vi "ADAM 5000 Get Voltages.vi"(8 "error in (no error)":errorcluster, 10 "AI Sensor Data":T1={"Sensor Array"=[{"Description"="P2 - LOX Tank Pressure", "Last Reading"="-124.89", "Coefs"=[-124.82, 244.17], "Eng Units"="psig"}, {"Description"="P3 - Fuel Tank Pressure", "Last Reading"="-124.89", "Coefs"=[-124.82, 244.17], "Eng Units"="psig"}, {"Description"="P1 - Chamber Pressure", "Last Reading"="-63.46", "Coefs"=[-63.442, 124.53], "Eng Units"="psig"}, {"Description"="Not Used", "Last Reading"="0.00", "Coefs"=[0.0, 0.0], "Eng Units"="psig"}, {"Description"="P5- DOME Reg.", "Last Reading"="-65.11", "Coefs"=[-65.132, -121.72], "Eng Units"="psig"}, {"Description"="Not Use", "Last Reading"="0.00", "Coefs"=[0.0, 0.0], "Eng Units"="psig"}, {"Description"="Load Cell", "Last Reading"="-6.72", "Coefs"=[-8.51, -8297.0], "Eng Units"="lb"}, {"Description"="P7 - Gnd High Pressure", "Last Reading"="-2.33", "Coefs"=[0.0, 10000.0], "Eng Units"="psig"}, {"Description"="High Press PT", "Last Reading"="-475.05", "Coefs"=[-483.6, 1244.5], "Eng Units"="psig"}, {"Description"="Dome Reg PT", "Last Reading"="-125.68", "Coefs"=[-126.9, 250.13], "Eng Units"="psig"}, {"Description"="FUEL PT", "Last Reading"="-125.44", "Coefs"=[-126.89, 250.01], "Eng Units"=""}, {"Description"="LOX PT", "Last Reading"="-128.32", "Coefs"=[-129.55, 251.63], "Eng Units"=""}, {"Description"="Chamber PT", "Last Reading"="-62.72", "Coefs"=[-63.442, 124.53], "Eng Units"=""}, {"Description"="LOX MV PT", "Last Reading"="-63.10", "Coefs"=[-63.711, 124.59], "Eng Units"=""}, {"Description"="FUEL MV PT", "Last Reading"="-61.90", "Coefs"=[-62.615, 123.79], "Eng Units"=""}, {"Description"="", "Last Reading"="0.00", "Coefs"=[0.0, 0.0], "Eng Units"=""}, {"Description"="Load Cell 0", "Last Reading"="-17.61", "Coefs"=[0.0, 16730.0], "Eng Units"=""}, {"Description"="Load Cell 1", "Last Reading"="13.17", "Coefs"=[0.0, 16730.0], "Eng Units"=""}, {"Description"="Load Cell 3", "Last Reading"="7.43", "Coefs"=[0.0, 16730.0], "Eng Units"=""}, {"Description"="Main Valve Closed Indicator", "Last Reading"="-0.00", "Coefs"=[0.0, 1.0], "Eng Units"="On/Off"}, {"Description"="Load Cell 1 - Veh Gross Weight", "Last Reading"="-125.78", "Coefs"=[-122.0, 8333.3], "Eng Units"="lbf"}, {"Description"="Load Cell 2 - - Veh Gross Weight", "Last Reading"="-3.62", "Coefs"=[0.0, 8333.33], "Eng Units"="lbf"}, {"Description"="Extra PT", "Last Reading"="-72.30", "Coefs"=[-72.241, 126.92], "Eng Units"=""}, {"Description"="Not Used", "Last Reading"="0.00", "Coefs"=[0.0, 0.0], "Eng Units"=""}, {"Description"="P6 - GHE Fill Pressure", "Last Reading"="-1035.38", "Coefs"=[-1035.0, 1261.6], "Eng Units"="psi"}, {"Description"="", "Last Reading"="0.00", "Coefs"=[], "Eng Units"=""}, {"Description"="", "Last Reading"="0.00", "Coefs"=[], "Eng Units"=""}, {"Description"="", "Last Reading"="0.00", "Coefs"=[], "Eng Units"=""}, {"Description"="", "Last Reading"="0.00", "Coefs"=[], "Eng Units"=""}, {"Description"="", "Last Reading"="0.00", "Coefs"=[], "Eng Units"=""}, {"Description"="", "Last Reading"="0.00", "Coefs"=[], "Eng Units"=""}, {"Description"="", "Last Reading"="0.00", "Coefs"=[], "Eng Units"=""}]}, 11 "Remote IP Address 2":string="192.168.10.200") -> (0 "error out":errorcluster, 1 "Slave Input Registers 2":u16[](array[numeric])=[32732, 32693, 32715, 32691, 32734, 32723, 32673, 32767] caption="Slave Input Registers (Read Only)", 2 "Master Raw Data Vdc":dbl[](array[numeric])=[-0.00016478571600001145, -0.00034331355899999493, -0.00024260554500000353, -0.0003524688330000174, -0.00015563044200001742, -0.0002059844489999989, -0.0004348662989999923, -4.568421000016088e-06], 3 "AI Sensor Data Out":T1={"Sensor Array"=[{"Description"="P2 - LOX Tank Pressure", "Last Reading"="-124.89", "Coefs"=[-124.82, 244.17], "Eng Units"="psig"}, {"Description"="P3 - Fuel Tank Pressure", "Last Reading"="-124.89", "Coefs"=[-124.82, 244.17], "Eng Units"="psig"}, {"Description"="P1 - Chamber Pressure", "Last Reading"="-63.46", "Coefs"=[-63.442, 124.53], "Eng Units"="psig"}, {"Description"="Not Used", "Last Reading"="0.00", "Coefs"=[0.0, 0.0], "Eng Units"="psig"}, {"Description"="P5- DOME Reg.", "Last Reading"="-65.10", "Coefs"=[-65.132, -121.72], "Eng Units"="psig"}, {"Description"="Not Use", "Last Reading"="0.00", "Coefs"=[0.0, 0.0], "Eng Units"="psig"}, {"Description"="Load Cell", "Last Reading"="-6.65", "Coefs"=[-8.51, -8297.0], "Eng Units"="lb"}, {"Description"="P7 - Gnd High Pressure", "Last Reading"="-2.43", "Coefs"=[0.0, 10000.0], "Eng Units"="psig"}, {"Description"="High Press PT", "Last Reading"="-476.38", "Coefs"=[-483.6, 1244.5], "Eng Units"="psig"}, {"Description"="Dome Reg PT", "Last Reading"="-125.68", "Coefs"=[-126.9, 250.13], "Eng Units"="psig"}, {"Description"="FUEL PT", "Last Reading"="-125.44", "Coefs"=[-126.89, 250.01], "Eng Units"=""}, {"Description"="LOX PT", "Last Reading"="-128.32", "Coefs"=[-129.55, 251.63], "Eng Units"=""}, {"Description"="Chamber PT", "Last Reading"="-62.72", "Coefs"=[-63.442, 124.53], "Eng Units"=""}, {"Description"="LOX MV PT", "Last Reading"="-63.10", "Coefs"=[-63.711, 124.59], "Eng Units"=""}, {"Description"="FUEL MV PT", "Last Reading"="-61.90", "Coefs"=[-62.615, 123.79], "Eng Units"=""}, {"Description"="", "Last Reading"="0.00", "Coefs"=[0.0, 0.0], "Eng Units"=""}, {"Description"="Load Cell 0", "Last Reading"="-17.61", "Coefs"=[0.0, 16730.0], "Eng Units"=""}, {"Description"="Load Cell 1", "Last Reading"="13.33", "Coefs"=[0.0, 16730.0], "Eng Units"=""}, {"Description"="Load Cell 2", "Last Reading"="7.43", "Coefs"=[0.0, 16730.0], "Eng Units"=""}, {"Description"="Main Valve Closed Indicator", "Last Reading"="-0.00", "Coefs"=[0.0, 1.0], "Eng Units"="On/Off"}, {"Description"="Load Cell 1 - Veh Gross Weight", "Last Reading"="-125.78", "Coefs"=[-122.0, 8333.3], "Eng Units"="lbf"}, {"Description"="Load Cell 2 - - Veh Gross Weight", "Last Reading"="-3.62", "Coefs"=[0.0, 8333.33], "Eng Units"="lbf"}, {"Description"="Extra PT", "Last Reading"="-72.30", "Coefs"=[-72.241, 126.92], "Eng Units"=""}, {"Description"="Not Used", "Last Reading"="0.00", "Coefs"=[0.0, 0.0], "Eng Units"=""}, {"Description"="P6 - GHE Fill Pressure", "Last Reading"="-1035.38", "Coefs"=[-1035.0, 1261.6], "Eng Units"="psi"}, {"Description"="", "Last Reading"="0.00", "Coefs"=[], "Eng Units"=""}, {"Description"="", "Last Reading"="0.00", "Coefs"=[], "Eng Units"=""}, {"Description"="", "Last Reading"="0.00", "Coefs"=[], "Eng Units"=""}, {"Description"="", "Last Reading"="0.00", "Coefs"=[], "Eng Units"=""}, {"Description"="", "Last Reading"="0.00", "Coefs"=[], "Eng Units"=""}, {"Description"="", "Last Reading"="0.00", "Coefs"=[], "Eng Units"=""}, {"Description"="", "Last Reading"="0.00", "Coefs"=[], "Eng Units"=""}]}, 4 "Eng Data":dbl[](array[numeric]), 5 "Eng Data & Units":string[](array[string]))   [LabVIEW 2018]
uses:
  Adam Stuff/nimodbus121/71/vi.lib/NI Modbus.llb/MB Modbus Command.ctl
  Type Defs/Sensor Data.ctl
panel:
  out "Post conversion":dbl[](array[numeric])
  out "ADC Vdc":dbl
  out "Slot 3 Vdc":dbl[](array[numeric])
  out "Slot 2 Vdc":dbl[](array[numeric])
  out "Slot 1 Vdc":dbl[](array[numeric])
  out "Slot 0 Vdc":dbl[](array[numeric])=[-0.00016478571600001145, -0.00034331355899999493, -0.00024260554500000353, -0.0003524688330000174, -0.00015563044200001742, -0.0002059844489999989, -0.0004348662989999923, -4.568421000016088e-06]
  in  "Modbus Command":T2={"Function Code"=3, "Starting Address"=0, "Quantity"=32, "Data"=[], "Discrete"=[]} {"Function Code" items=["Read Coils"=1, "Read Discrete Inputs"=2, "Read Holding Registers"=3, "Read Input Registers"=4, "Write Single Coil"=5, "Write Single Register"=6, "Read Exception Status"=7, "Write Multiple Coils"=15, "Write Multiple Registers"=16]}
  in  "Remote Port 2":u16=502
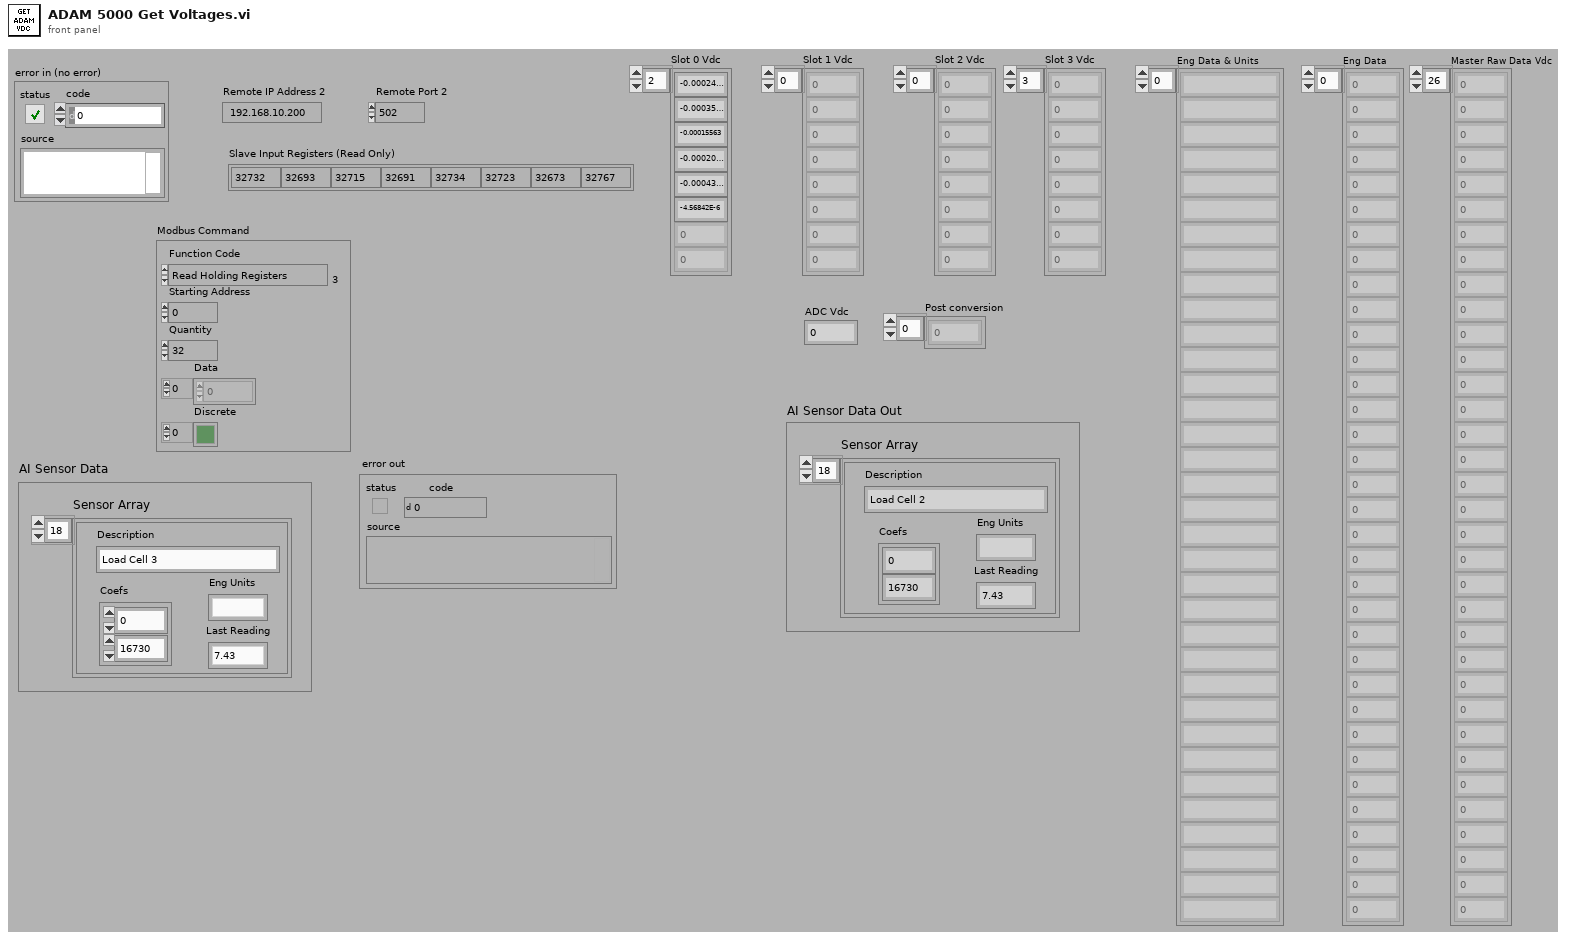
[diagram p1: front panel]
types:
  T1 = typedef "Sensor Data.ctl" = cluster{"Sensor Array":cluster{"Description":string, "Last Reading":string, "Coefs":dbl[], "Eng Units":string}[]}
  T2 = typedef "MB Modbus Command.ctl" = cluster{"Function Code":u8, "Starting Address":u16, "Quantity":u16, "Data":u16[], "Discrete":bool[]}
  T3 = cluster{"Description":string, "Last Reading":string, "Coefs":dbl[], "Eng Units":string}[]
  T4 = cluster{"Description":string, "Last Reading":string, "Coefs":dbl[], "Eng Units":string}
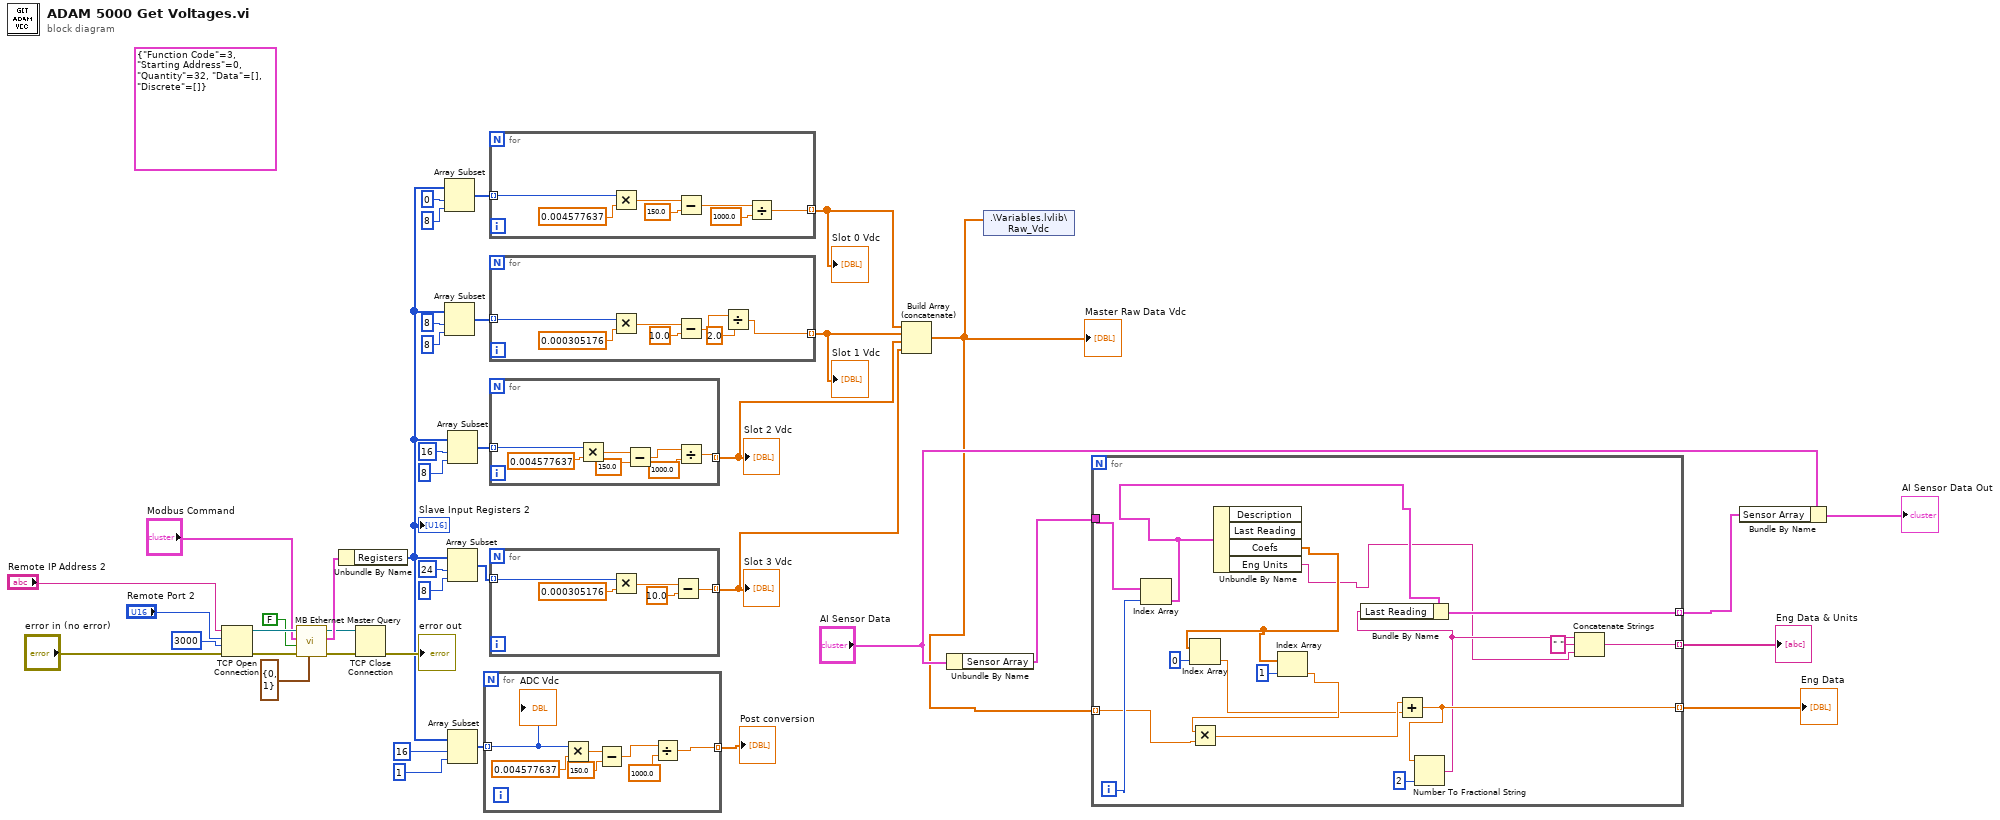
[diagram p0: block diagram]
diagram:
  (unwired) T2 {"Function Code"=3, "Starting Address"=0, "Quantity"=32, "Data"=[], "Discrete"=[]} ("Modbus Command")
  n1 = TCP Open Connection(address="Remote IP Address 2", remote port or service name="Remote Port 2", timeout ms (60000)=3000, error in (no error)="error in (no error)") -> (connection ID=w39:refnum<k5>, error out=w33:errorcluster)  [unwired: 1 in]
  n2 = call "MB Ethernet Master Query.vi"("MBAP Header"=cluster{"Transaction ID":u16, "Unit ID":u8} {"Transaction ID"=0, "Unit ID"=1}, "error in (no error)"=w33, "Use MODBUS Data Unit?"=FALSE, "Modbus Command"="Modbus Command", "TCP Connection Refnum in"=w39) -> ("error out"=w32:errorcluster, "Registers"=w37:cluster{"Registers":u16[], "Discrete":bool[]}, "TCP Connection Refnum (dup)"=w34:refnum<k5>)  [unwired: 2 in, 2 out]
  n3 = Unbundle By Name(w37) -> ("Registers"=w5:u16[])
  "Slave Input Registers 2" <- w5
  n4 = TCP Close Connection(connection ID=w34, error in (no error)=w32) -> (error out=→"error out":errorcluster)  [unwired: 1 in, 1 out]
  n5 = Array Subset(array=w5, index=0, length=8) -> (w26:u16[])
  n6 = Array Subset(array=w5, index=8, length=8) -> (w25:u16[])
  n7 = Array Subset(array=w5, index=16, length=8) -> (w20:u16[])
  n8 = Array Subset(array=w5, index=24, length=8) -> (w19:u16[])
  n9 = Array Subset(array=w5, index=16, length=1) -> (w6:u16[])
  n10 = for {
    tunnel: w6 -> [w45] mode=indexing
    tunnel: [w43] -> w2 mode=indexing
    n11 = Multiply(x=w45, y=0.004577637) -> (x*y=w47:dbl)
    n12 = Subtract(x=w47, y=150.0) -> (x-y=w44:dbl)
    n13 = Divide(x=w44, y=1000.0) -> (x/y=w43:dbl)
    "ADC Vdc" <- w45
  }
  "Post conversion" <- w2
  n14 = for {
    tunnel: w26 -> [w55] mode=indexing
    tunnel: [w49] -> w16 mode=indexing
    n15 = Multiply(x=w55, y=0.004577637) -> (x*y=w53:dbl)
    n16 = Subtract(x=w53, y=150.0) -> (x-y=w51:dbl)
    n17 = Divide(x=w51, y=1000.0) -> (x/y=w49:dbl)
  }
  "Slot 0 Vdc" <- w16
  n18 = for {
    tunnel: w25 -> [w62] mode=indexing
    tunnel: [w58] -> w15 mode=indexing
    n19 = Multiply(x=w62, y=0.000305176) -> (x*y=w60:dbl)
    n20 = Subtract(x=w60, y=10.0) -> (x-y=w56:dbl)
    n21 = Divide(x=w56, y=2.0) -> (x/y=w58:dbl)
  }
  "Slot 1 Vdc" <- w15
  n22 = for {
    tunnel: w20 -> [w69] mode=indexing
    tunnel: [w65] -> w14 mode=indexing
    n23 = Multiply(x=w69, y=0.004577637) -> (x*y=w68:dbl)
    n24 = Subtract(x=w68, y=150.0) -> (x-y=w63:dbl)
    n25 = Divide(x=w63, y=1000.0) -> (x/y=w65:dbl)
  }
  "Slot 2 Vdc" <- w14
  n26 = for {
    tunnel: w19 -> [w74] mode=indexing
    tunnel: [w70] -> w13 mode=indexing
    n27 = Multiply(x=w74, y=0.000305176) -> (x*y=w72:dbl)
    n28 = Subtract(x=w72, y=10.0) -> (x-y=w70:dbl)
  }
  "Slot 3 Vdc" <- w13
  n29 = Build Array (concatenate)(w16, w15, w14, w13) -> (w1:dbl[])
  "Master Raw Data Vdc" <- w1
  n30 = Unbundle By Name("AI Sensor Data") -> ("Sensor Array"=w12:T3)
  n31 = shared-variable ".\\Variables.lvlib\\Raw_Vdc"(w1) -> ()  [unwired: 1 in, 1 out]
  n32 = for {
    tunnel: w12 -> [w91]
    tunnel: w1 -> [w85] mode=indexing
    tunnel: [w81] -> w11 mode=indexing
    tunnel: [w79] -> w9 mode=indexing
    tunnel: [w75] -> w7 mode=indexing
    i -> [w90]
    n33 = Index Array(array=w91, index=w90) -> (element=w89:T4)
    n34 = Unbundle By Name(w89) -> ("Coefs"=w86:dbl[], "Eng Units"=w76:string)  [unwired: 2 out]
    n35 = Index Array(array=w86, index=0) -> (element=w82:dbl)
    n36 = Index Array(array=w86, index=1) -> (element=w84:dbl)
    n37 = Multiply(x=w84, y=w85) -> (x*y=w83:dbl)
    n38 = Add(x=w83, y=w82) -> (x+y=w81:dbl)
    n39 = Number To Fractional String(number=w81, precision (6)=i16 2) -> (F-format string=w78:string)  [unwired: 2 in]
    n40 = Bundle By Name(cluster=w89, "Last Reading"=w78) -> (w79:T4)
    n41 = Concatenate Strings(w78, " " ("string"), w76) -> (w75:string)
  }
  "Eng Data" <- w11
  "Eng Data & Units" <- w7
  n42 = Bundle By Name(cluster="AI Sensor Data", "Sensor Array"=w9) -> (→"AI Sensor Data Out":T1)
